vi "Configure FFT Measurement Peak Search.vi"(6 "To":dbl[](array[numeric]) format="%^.3e", 7 "From":dbl[](array[numeric]) format="%^.3e", 8 "error in (no error)":errorcluster, 9 "Enable Full Span":bool[](array[boolean]), 10 "Instance (1)":i32=1, 11 "VISA resource name":refnum<visa-resource-name>) -> (0 "error out":errorcluster, 3 "VISA resource name out":refnum<visa-resource-name>)   [LabVIEW 2020, in "Rohde&Schwarz CMXP GPRF.lvlib"]
doc: "Defines the peak search ranges. The search ranges are automatically adjusted if the frequency span fs is reduced (CONFigure:GPRF:MEAS<i>:FFTSanalyzer:FSPan).\n\nAttribute:\nRSCMXPGPRF_ATTR_FFT_MEASUREMENT_PEAK_SEARCH\n\nRemote-control command:\nCONFigure:GPRF:MEAS<i>:FFTSanalyzer:PSEarch"
uses:
  <instrlib>/Rohde&Schwarz CMXP GPRF/Rohde&Schwarz CMXP GPRF.lvlib
  <instrlib>/Rohde&Schwarz CMXP GPRF/Private/rsidr_core.llb/rsidr_core.lvlib
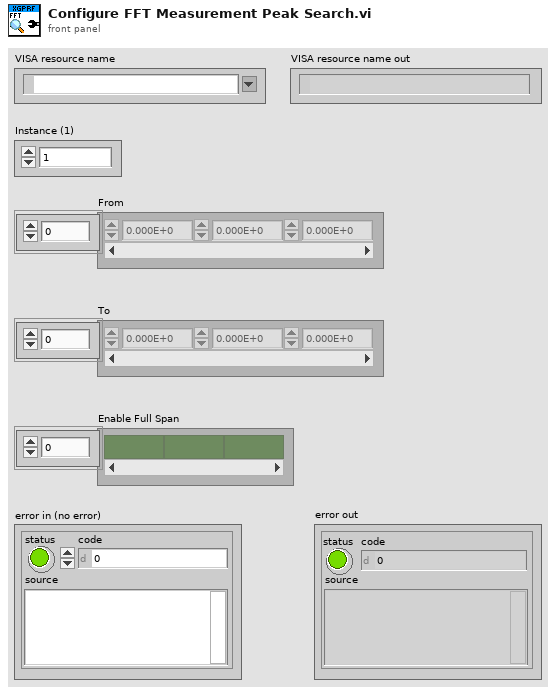
[diagram p1: front panel]
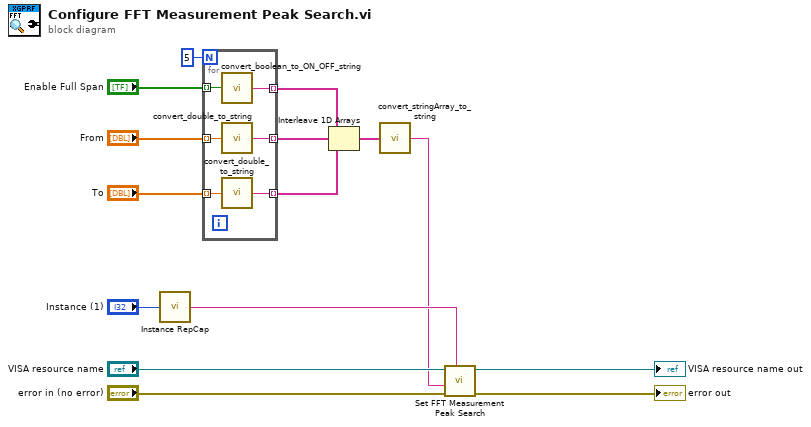
[diagram p0: block diagram]
diagram:
  n1 = call <instrlib>:"Instance RepCap.vi"("Instance in"="Instance (1)") -> ("Instance out"=w6:string)
  n2 = for {
    N: 5 -> [_]
    tunnel: "Enable Full Span" -> [w20] mode=indexing
    tunnel: [w21] -> w13 mode=indexing
    tunnel: "From" -> [w19] mode=indexing
    tunnel: "To" -> [w18] mode=indexing
    tunnel: [w17] -> w2 mode=indexing
    tunnel: [w16] -> w1 mode=indexing
    n3 = call <instrlib>:"convert_boolean_to_ON_OFF_string.vi"("boolean value in"=w20) -> ("string value out"=w21:string)  [unwired: 4 in]
    n4 = call <instrlib>:"convert_double_to_string.vi"("double in"=w19) -> ("string out"=w17:string)  [unwired: 4 in]
    n5 = call <instrlib>:"convert_double_to_string.vi"("double in"=w18) -> ("string out"=w16:string)  [unwired: 4 in]
  }
  n6 = Interleave 1D Arrays(w13, w2, w1) -> (w12:string[])
  n7 = call <instrlib>:"convert_stringArray_to_string.vi"("string array in"=w12) -> ("string out"=w5:string)  [unwired: 4 in]
  n8 = call "Set FFT Measurement Peak Search"("Repeated Capabilities"=w6, "error in (no error)"="error in (no error)", "FFT Measurement Peak Search ()"=w5, "instrument handle"="VISA resource name") -> ("error out"=→"error out":errorcluster, "instrument handle out"=→"VISA resource name out":refnum<visa-resource-name>)  [unwired: 6 in]
